vi "MailMonitor.vi"() -> ()   [LabVIEW 2025]
uses:
  <userlib>/_OpenG.lib/comparison/comparison.llb/I32 Changed__ogtk.vi
  <vilib>/smtpClient/Set Message Text.vi
  <vilib>/smtpClient/LabVIEWSMTPClient.lvlib
  <userlib>/_OpenG.lib/comparison/comparison.llb/openg_comparison__ogtk.lvlib
panel:
  in  "LogFile":path
  in  "stop":bool
  in  "Recipients":string[](array[string])=["dpl@aber.ac.uk"]
  in  "TVC_CyclesRemaining":i32=1
  in  "TVC_CycleNumber":i32
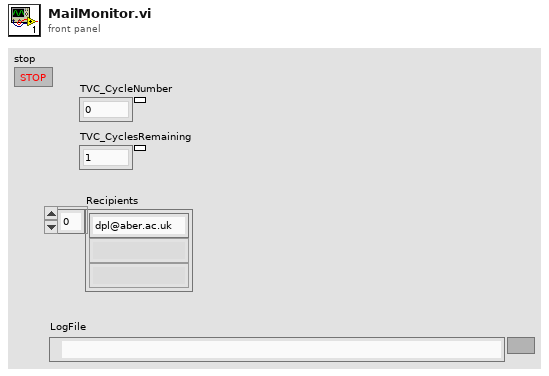
[diagram p1: front panel]
types:
  T1 = typedef "LabVIEWSMTPClient.lvlib/SmtpClientHandle.ctl" = refnum<k1>
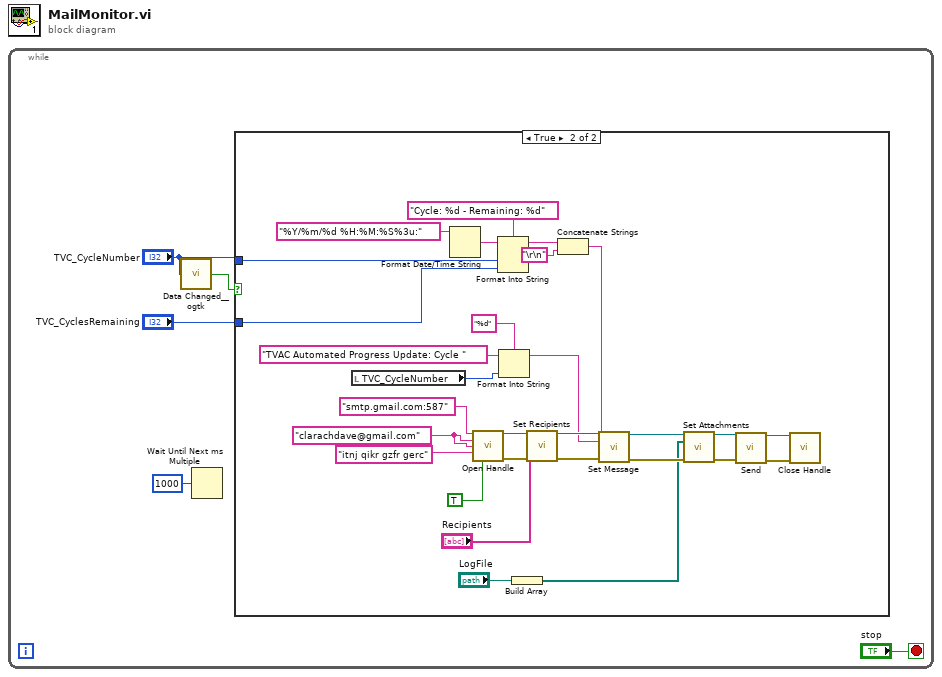
[diagram p0: block diagram]
diagram:
  n1 = while {
    stop <- "stop" stop-if-true
    n2 = call-poly <userlib>:"Data Changed__ogtk.vi"("I32"="TVC_CycleNumber") -> ("Changed"=w1:bool)
    n3 = Wait Until Next ms Multiple(millisecond multiple=u32 1000) -> ()  [unwired: 1 out]
    n4 = case shown="True" w1 {
      tunnel: "TVC_CycleNumber" -> [_ w16]
      tunnel: "TVC_CyclesRemaining" -> [_ w15]
      frame False {
      }
      frame True {
        w24 = "clarachdave@gmail.com" ("from")
        n5 = local read "TVC_CycleNumber"() -> (w21:i32)
        n6 = Format Date/Time String(time format string (%c)="%Y/%m/%d %H:%M:%S%3u:") -> (date/time string=w18:string)  [unwired: 2 in]
        n7 = call <vilib>:"Open Handle.vi"("server address"="smtp.gmail.com:587", "from"=w24, "username"=w24, "password"="itnj qikr gzfr gerc", "use TLS (false)"=TRUE) -> ("handle out"=w32:T1, "error out"=w31:errorcluster)  [unwired: 9 in]
        n8 = Format Into String(format string="Cycle: %d - Remaining: %d", initial string=w18, w16, w15) -> (resulting string=w14:string)  [unwired: 1 in, 1 out]
        n9 = Format Into String(format string="%d", initial string="TVAC Automated Progress Update: Cycle " ("subject"), w21) -> (resulting string=w20:string)  [unwired: 1 in, 1 out]
        n10 = Build Array("LogFile") -> (w6:path[])
        n11 = call <vilib>:"Set Recipients.vi"("handle in"=w32, "to"="Recipients", "error in (no error)"=w31) -> ("handle out"=w29:T1, "error out"=w28:errorcluster)  [unwired: 11 in]
        n12 = Concatenate Strings(w14, "\r\n") -> (w12:string)
        n13 = call-poly <vilib>:"Set Message.vi"("handle in"=w29, "subject"=w20, "plain text message"=w12, "error in (no error)"=w28) -> ("handle out"=w10:T1, "error out"=w9:errorcluster)  [unwired: 10 in]
        n14 = call <vilib>:"Set Attachments.vi"("handle in"=w10, "attachments"=w6, "error in (no error)"=w9) -> ("handle out"=w11:T1, "error out"=w8:errorcluster)  [unwired: 11 in]
        n15 = call <vilib>:"Send.vi"("handle in"=w11, "error in (no error)"=w8) -> ("handle out"=w27:T1, "error out"=w26:errorcluster)  [unwired: 11 in, 1 out]
        n16 = call <vilib>:"Close Handle.vi"("handle in"=w27, "error in (no error)"=w26) -> ()  [unwired: 12 in, 2 out]
      }
    }
  }
